vi "Get Fit Values.vi"(8 "error in (no error)":errorcluster, 11 "Head Impulse Fit in":refnum<class "Head Impulse Fit.lvclass">) -> (0 "error out":errorcluster, 2 "Fit Data":T1 {"Window Eye Lag (ms)" format="%#_4g"; "Window Gain" format="%#_4g"}, 3 "Head Impulse Fit out":refnum<class "Head Impulse Fit.lvclass">)   [LabVIEW 2014, in "Head Impulse Fit.lvclass"]
uses:
  Head Impulse Fit.lvclass
  Fit Data.ctl
  Head Impulse Fit.lvclass/Head Impulse Fit.ctl
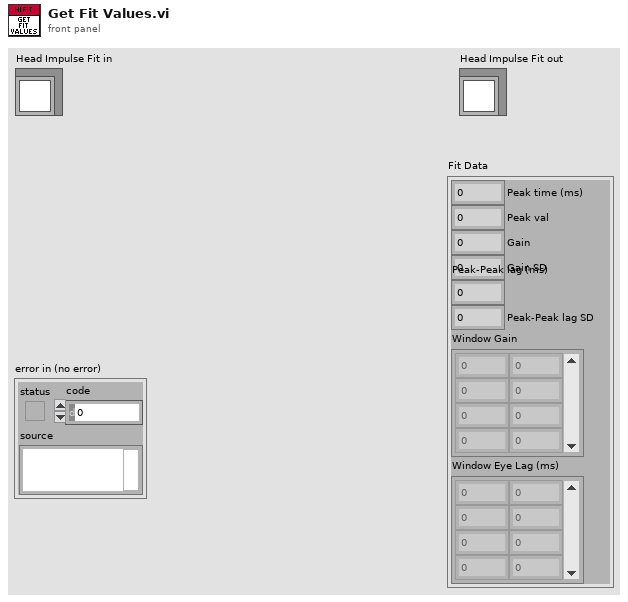
[diagram p1: front panel]
types:
  T1 = typedef "Head Impulse Fit.lvclass/Fit Data.ctl" = cluster{"Peak time (ms)":dbl, "Peak val":dbl, "Gain":dbl, "Gain SD":dbl, "Peak-Peak lag (ms)":dbl, "Peak-Peak lag SD":dbl, "Window Gain":dbl[][], "Window Eye Lag (ms)":dbl[][]}
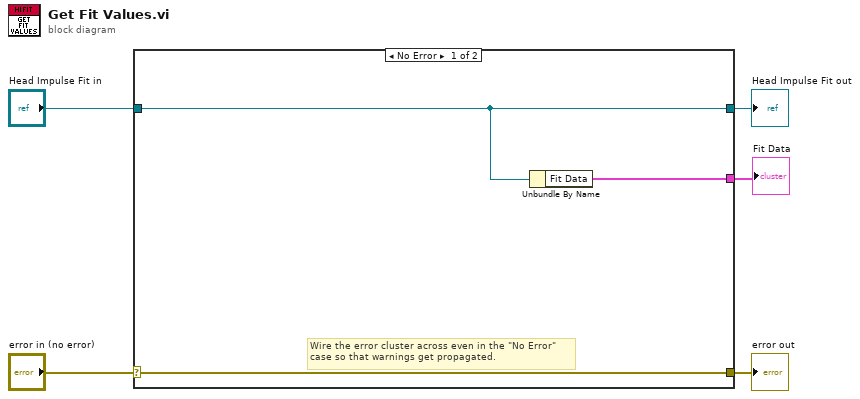
[diagram p0: block diagram]
diagram:
  n1 = case shown="No Error" "error in (no error)" {
    selector: "error in (no error)" -> [w8 w10]
    tunnel: [w8 w10] -> w4
    tunnel: [w7 w9] -> w2
    tunnel: "Head Impulse Fit in" -> [w7 w9]
    tunnel: [w6 _] -> w1
    frame No Error {
      # "Wire the error cluster across even in the \"No Error\"\ncase so that warnings get propagated."
      n2 = Unbundle By Name(w7) -> ("Fit Data"=w6:T1)
    }
    frame Error {
    }
  }
  "error out" <- w4
  "Head Impulse Fit out" <- w2
  "Fit Data" <- w1
